vi "Content.vi"(7 "Context":refnum<class "Context.lvclass">, 8 "Error In":errorcluster, 11 "Abstract In":refnum<class "Abstract.lvclass">) -> (0 "Error Out":errorcluster, 2 "Content":string, 3 "Abstract Out":refnum<class "Abstract.lvclass">)   [LabVIEW 2018, in "Toolkit.lvlib" / "Nodes.lvlib" / "Abstract.lvclass"]
uses:
  Abstract.lvclass
  Data/Context/Context.lvclass
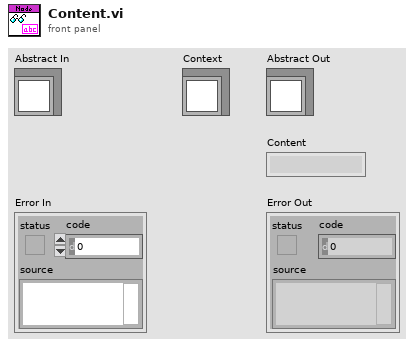
[diagram p1: front panel]
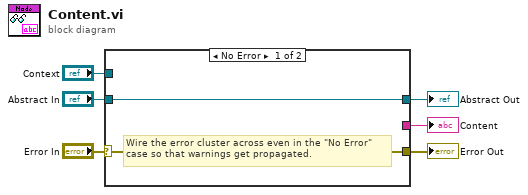
[diagram p0: block diagram]
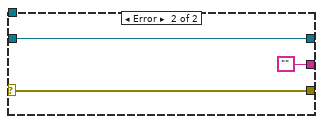
[diagram p2: hidden frame]
diagram:
  n1 = case shown="No Error" "Error In" {
    selector: "Error In" -> [w7 w11]
    tunnel: [w7 w11] -> w5
    tunnel: [w8 w10] -> w3
    tunnel: "Abstract In" -> [w8 w10]
    tunnel: [_ ""] -> w2
    tunnel: "Context" -> [_ _]
    frame No Error {
      # "Wire the error cluster across even in the \"No Error\"\ncase so that warnings get propagated."
    }
    frame Error {
    }
  }
  "Error Out" <- w5
  "Abstract Out" <- w3
  "Content" <- w2
